vi "balloon入队列.vi"(7 "队列":refnum<queue>, 9 "告警信息":string, 10 "故障信息":string) -> (3 "队列输出":refnum<queue>)   [LabVIEW 2016]
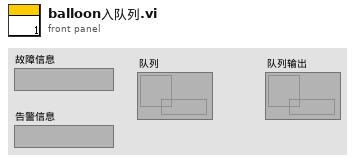
[diagram p1: front panel]
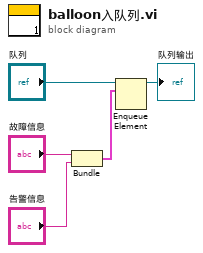
[diagram p0: block diagram]
diagram:
  n1 = Bundle("故障信息"="故障信息", "告警信息"="告警信息") -> (w5:cluster{"故障信息":string, "告警信息":string})  [unwired: 1 in]
  n2 = Enqueue Element(queue="队列", element=w5) -> (queue out=→"队列输出":refnum<queue>)  [unwired: 2 in, 2 out]
